vi "Update Cyclic_Status.vi"(8 "error in (no error)":errorcluster, 11 "DUT Sample in":refnum<class "DUT Sample.lvclass">) -> (0 "error out":errorcluster, 3 "DUT Sample out":refnum<class "DUT Sample.lvclass">)   [LabVIEW 2023, in "DUT Sample.lvclass"]
uses:
  DUT Sample.lvclass
  DUT Sample.lvclass/DUT Sample.ctl
  <vilib>/xnet/xnet.llb/XNET Write (Signal Single-point).vi
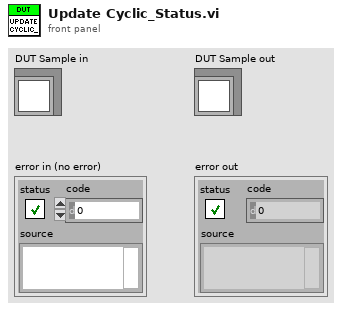
[diagram p1: front panel]
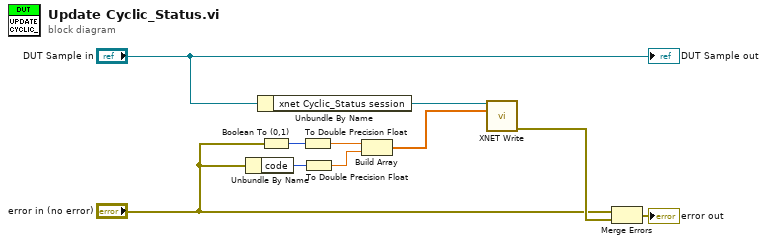
[diagram p0: block diagram]
diagram:
  n1 = Unbundle By Name("error in (no error)") -> ("code"=w1:i32)
  n2 = Unbundle By Name("DUT Sample in") -> ("xnet Cyclic_Status session"=w9:refnum<k21>)
  n3 = Boolean To (0,1)(Boolean="error in (no error)") -> (0, 1=w8:i16)
  n4 = To Double Precision Float(number=w8) -> (double precision float=w7:dbl)
  n5 = To Double Precision Float(number=w1) -> (double precision float=w6:dbl)
  n6 = Build Array(w7, w6) -> (w5:dbl[])
  n7 = call-poly <vilib>:"XNET Write.vi"("session in"=w9, "data"=w5) -> ("error out"=w3:errorcluster)  [unwired: 12 in, 1 out]
  n8 = Merge Errors("error in (no error)", w3) -> (→"error out":errorcluster)
  "DUT Sample out" <- "DUT Sample in"
